vi "Inner Loop Control Select.vi"(8 "Controller - User Input":T2={"Num Inner Loop"=[-11.0745, 19.702, -8.7598], "Den Inner Loop"=[1.0, -1.49756, 0.49756], "Inner Loop Gain"=1.0, "IMU_sample_rate"=0, "Num Outer Loop"=[0.1636, -0.16289, 0.0], "Den Outer Loop"=[1.0, -0.6326, 0.0], "Outer Loop Gain"=1.0, "Outer Loop sample rate"=20.0}, 11 "Controller Select":T1(ring)=enum."100hz/100hz" caption="Enum") -> (0 "Inner Loop Controller":T3, 4 "Outer Loop sample rate out":dbl)   [LabVIEW 2014]
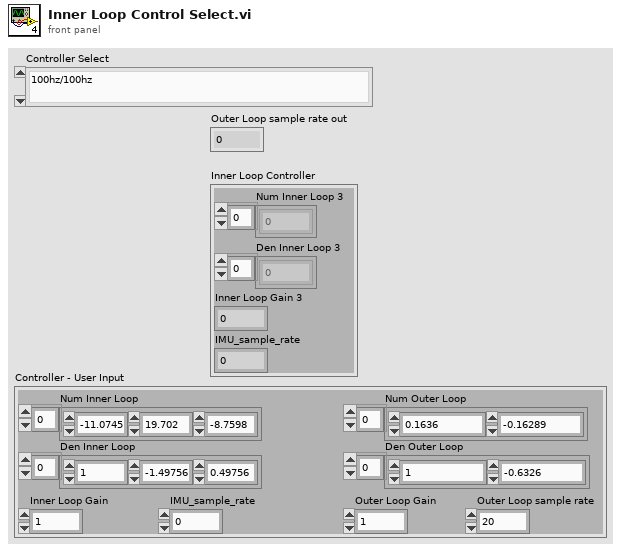
[diagram p1: front panel]
types:
  T1 = enum16{"100hz/50hz", "100hz/100hz", "200hz/200hz", "200hz/20hz", "User Defined"}
  T2 = cluster{"Num Inner Loop":dbl[], "Den Inner Loop":dbl[], "Inner Loop Gain":dbl, "IMU_sample_rate":i32, "Num Outer Loop":dbl[], "Den Outer Loop":dbl[], "Outer Loop Gain":dbl, "Outer Loop sample rate":dbl}
  T3 = cluster{"Num Inner Loop 3":dbl[], "Den Inner Loop 3":dbl[], "Inner Loop Gain 3":dbl, "IMU_sample_rate":i32}
  T4 = cluster{"Num Inner Loop":dbl[], "Den Inner Loop":dbl[], "Inner Loop Gain":dbl, "IMU_sample_rate":i32}
  T5 = cluster{"Num Inner Loop 3":dbl[], "Den Inner Loop 3":dbl[], "Inner Loop Gain 3":dbl, i32}
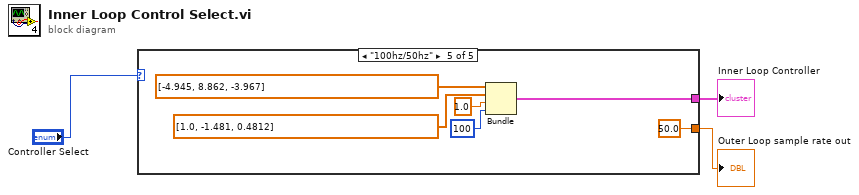
[diagram p0: block diagram]
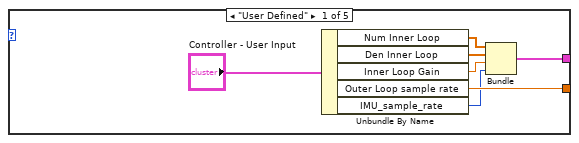
[diagram p2: hidden frame]
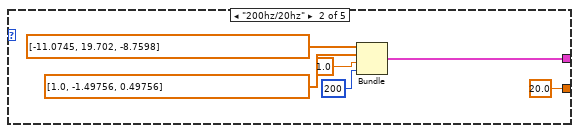
[diagram p3: hidden frame]
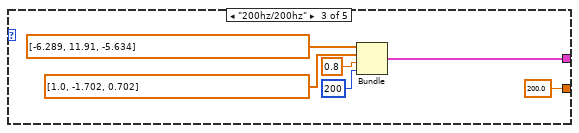
[diagram p4: hidden frame]
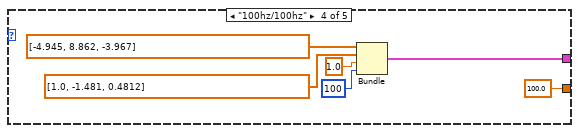
[diagram p5: hidden frame]
diagram:
  n1 = case shown="\"100hz/50hz\"" "Controller Select" {
    tunnel: [w10 20.0 ("Outer Loop sample rate") 200.0 ("Outer Loop sample rate") 100.0 ("Outer Loop sample rate") 50.0 ("Outer Loop sample rate")] -> w3
    tunnel: [w6 w12 w18 w24 w30] -> w2
    frame "User Defined" {
      n2 = Unbundle By Name("Controller - User Input") -> ("Num Inner Loop"=w9:dbl[], "Den Inner Loop"=w8:dbl[], "Inner Loop Gain"=w7:dbl, "Outer Loop sample rate"=w10:dbl, "IMU_sample_rate"=w5:i32)
      n3 = Bundle("Num Inner Loop"=w9, "Den Inner Loop"=w8, "Inner Loop Gain"=w7, "IMU_sample_rate"=w5) -> (w6:T4)  [unwired: 1 in]
    }
    frame "200hz/20hz" {
      n4 = Bundle("Num Inner Loop 3"=dbl[] [-11.0745, 19.702, -8.7598], "Den Inner Loop 3"=dbl[] [1.0, -1.49756, 0.49756], "Inner Loop Gain 3"=1.0, 200) -> (w12:T5)  [unwired: 1 in]
    }
    frame "200hz/200hz" {
      n5 = Bundle("Num Inner Loop 3"=dbl[] [-6.289, 11.91, -5.634], "Den Inner Loop 3"=dbl[] [1.0, -1.702, 0.702], "Inner Loop Gain 3"=0.8, 200) -> (w18:T5)  [unwired: 1 in]
    }
    frame "100hz/100hz" {
      n6 = Bundle("Num Inner Loop 3"=dbl[] [-4.945, 8.862, -3.967], "Den Inner Loop 3"=dbl[] [1.0, -1.481, 0.4812], "Inner Loop Gain 3"=1.0, 100) -> (w24:T5)  [unwired: 1 in]
    }
    frame "100hz/50hz" {
      n7 = Bundle("Num Inner Loop 3"=dbl[] [-4.945, 8.862, -3.967], "Den Inner Loop 3"=dbl[] [1.0, -1.481, 0.4812], "Inner Loop Gain 3"=1.0, 100) -> (w30:T5)  [unwired: 1 in]
    }
  }
  "Outer Loop sample rate out" <- w3
  "Inner Loop Controller" <- w2
